vi "反控数据上传(子VI).vi"(11 "QN":string) -> ()   [LabVIEW 2016, in "数据传输系统.lvlib"]
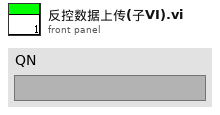
[diagram p1: front panel]
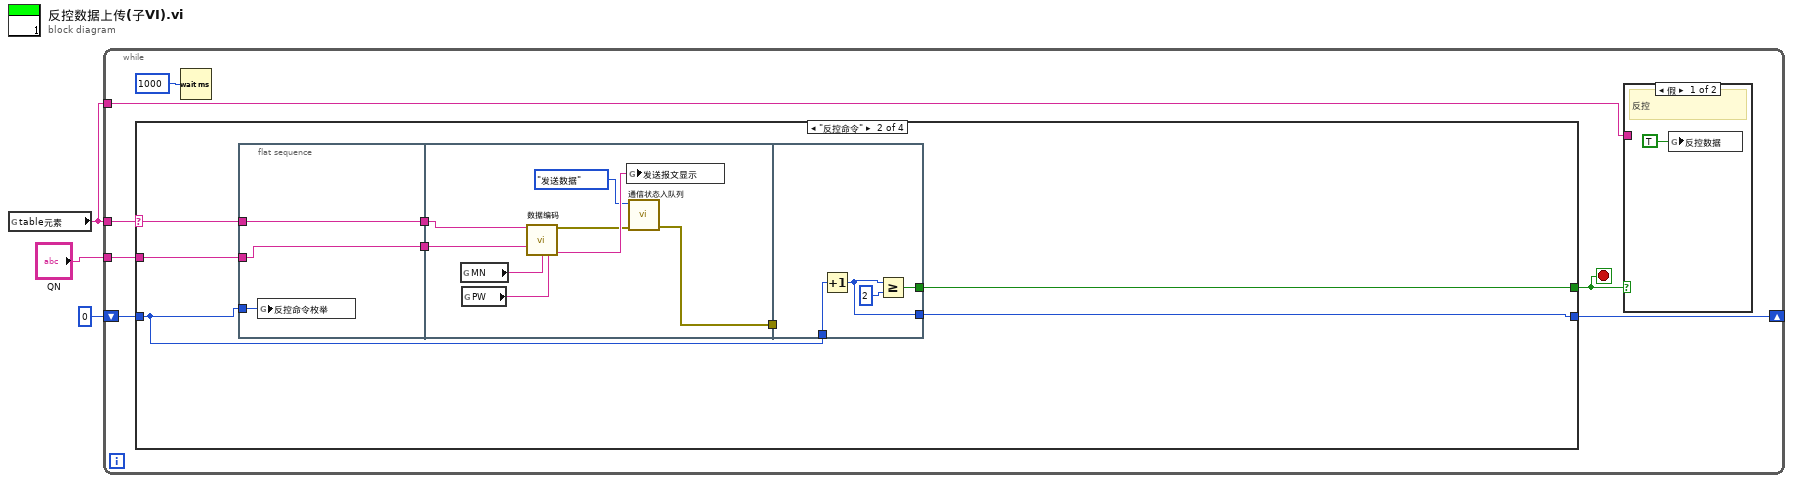
[diagram p0: block diagram]
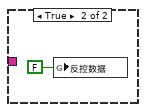
[diagram p2: hidden frame]
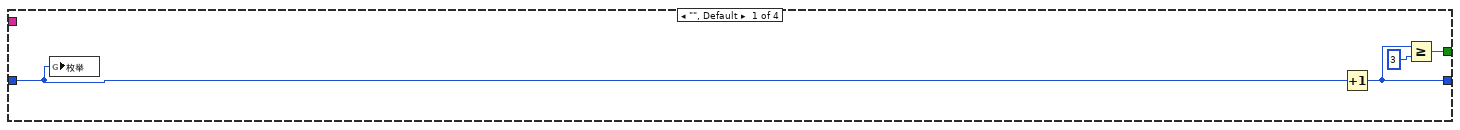
[diagram p3: hidden frame]
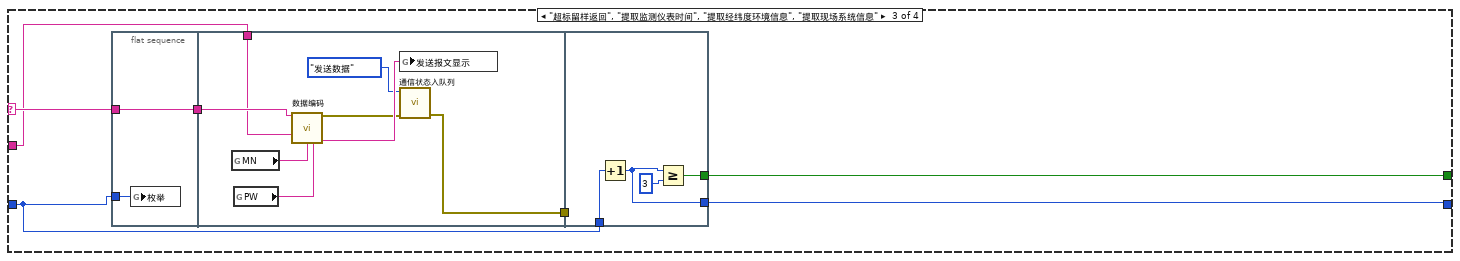
[diagram p4: hidden frame]
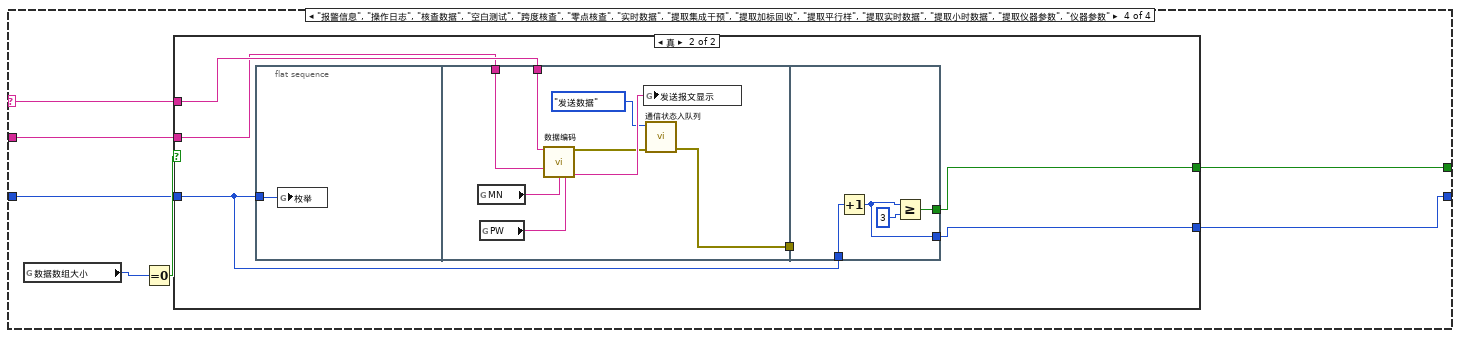
[diagram p5: hidden frame]
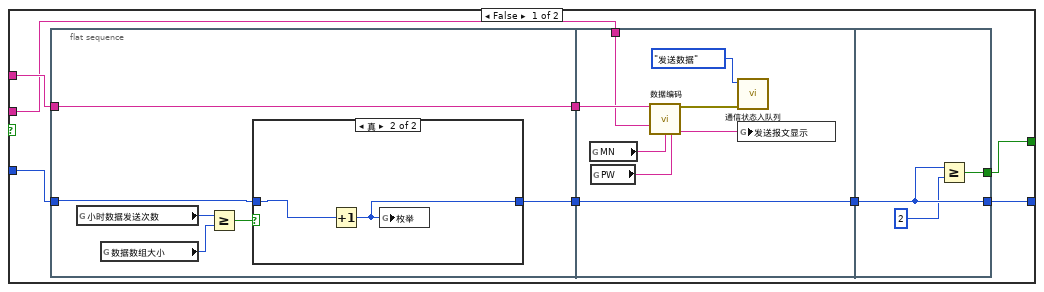
[diagram p6: hidden frame]
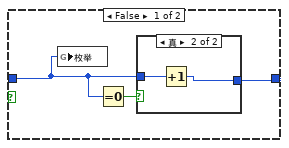
[diagram p7: hidden frame]
diagram:
  n1 = global read "全局1.vi" "table元素"() -> (w3:string)
  n2 = while {
    tunnel: w3 -> [w10]
    shift-right: [w8] -> _
    shift-left: 0 -> [w9]
    tunnel: w3 -> [w6]
    tunnel: "QN" -> [w4]
    stop <- w7 stop-if-true
    n3 = case shown="\"反控命令\"" w10 {
      selector: w10 -> [_ w21 w46 w63]
      tunnel: w9 -> [w15 w22 w43 w62]
      tunnel: [w14 w19 w42 w67] -> w7
      tunnel: [w13 w20 w41 w66] -> w8
      tunnel: w4 -> [_ w18 w40 w61]
      frame "", Default {
        n4 = global write "全局1.vi" "枚举"(w15) -> ()
        n5 = Increment(x=w15) -> (x+1=w13:i32)
        n6 = Greater Or Equal?(x=w13, y=3) -> (x >= y?=w14:bool)
      }
      frame "反控命令" {
        n7 = flat-sequence {
          tunnel: w21 -> [w27]
          tunnel: [w27] -> w24
          tunnel: w22 -> [w26]
          tunnel: w18 -> [w25]
          tunnel: [w25] -> w17
          tunnel: w24 -> [w30]
          tunnel: [w29] -> w23
          tunnel: w17 -> [w28]
          tunnel: w23 -> [_]
          tunnel: w22 -> [w38]
          tunnel: [w37] -> w19
          tunnel: [w36] -> w20
          frame #0 {
            n8 = global write "全局 反控命令枚举.vi" "反控命令枚举"(w26) -> ()
          }
          frame #1 {
            n9 = global read "断电保存全局.vi" "MN"() -> (w35:string)
            n10 = global read "断电保存全局.vi" "PW"() -> (w34:string)
            n11 = call "数据编码.vi"("table输入"=w30, "QN"=w28, "MN"=w35, "PW"=w34) -> ("错误常量"=w32:errorcluster, "通讯包字符串"=w33:string)  [unwired: 10 in]
            n12 = global write "全局1.vi" "发送报文显示"(w33) -> ()
            n13 = call "通信状态入队列.vi"("错误输入（无错误）"=w32, "枚举"=enum16{"打开连接", "发送数据", "读取数据", "数据处理", "关闭连接"}."发送数据") -> ("错误输出"=w29:errorcluster)  [unwired: 9 in]
          }
          frame #2 {
            n14 = Increment(x=w38) -> (x+1=w36:i32)
            n15 = Greater Or Equal?(x=w36, y=2) -> (x >= y?=w37:bool)
          }
        }
      }
      frame "超标留样返回", "提取监测仪表时间", "提取经纬度环境信息", "提取现场系统信息" {
        n16 = flat-sequence {
          tunnel: w46 -> [w48]
          tunnel: [w48] -> w45
          tunnel: w43 -> [w47]
          tunnel: w45 -> [w51]
          tunnel: [w50] -> w44
          tunnel: w40 -> [w49]
          tunnel: w44 -> [_]
          tunnel: w43 -> [w59]
          tunnel: [w58] -> w42
          tunnel: [w57] -> w41
          frame #0 {
            n17 = global write "全局1.vi" "枚举"(w47) -> ()
          }
          frame #1 {
            n18 = global read "断电保存全局.vi" "MN"() -> (w56:string)
            n19 = global read "断电保存全局.vi" "PW"() -> (w55:string)
            n20 = call "数据编码.vi"("table输入"=w51, "QN"=w49, "MN"=w56, "PW"=w55) -> ("错误常量"=w53:errorcluster, "通讯包字符串"=w54:string)  [unwired: 10 in]
            n21 = global write "全局1.vi" "发送报文显示"(w54) -> ()
            n22 = call "通信状态入队列.vi"("错误输入（无错误）"=w53, "枚举"=enum16{"打开连接", "发送数据", "读取数据", "数据处理", "关闭连接"}."发送数据") -> ("错误输出"=w50:errorcluster)  [unwired: 9 in]
          }
          frame #2 {
            n23 = Increment(x=w59) -> (x+1=w57:i32)
            n24 = Greater Or Equal?(x=w57, y=3) -> (x >= y?=w58:bool)
          }
        }
      }
      frame "报警信息", "操作日志", "核查数据", "空白测试", "跨度核查", "零点核查", "实时数据", "提取集成干预", "提取加标回收", "提取平行样", "提取实时数据", "提取小时数据", "提取仪器参数", "仪器参数" {
        n25 = global read "全局 数据数组大小.vi" "数据数组大小"() -> (w65:i32)
        n26 = Equal To 0?(x=w65) -> (x = 0?=w64:bool)
        n27 = case shown="真" w64 {
          tunnel: [w72 w102] -> w67
          tunnel: [w71 w103] -> w66
          tunnel: w63 -> [w70 w105]
          tunnel: w62 -> [w69 w104]
          tunnel: w61 -> [w68 w101]
          frame False {
            n28 = flat-sequence {
              tunnel: w69 -> [w78]
              tunnel: [w76] -> w75
              tunnel: w70 -> [w77]
              tunnel: [w77] -> w74
              tunnel: w75 -> [w97]
              tunnel: [w97] -> w73
              tunnel: w74 -> [w91]
              tunnel: w68 -> [w90]
              tunnel: w73 -> [w100]
              tunnel: [w100] -> w71
              tunnel: [w99] -> w72
              frame #0 {
                n29 = global read "全局 小时数据发送次数.vi" "小时数据发送次数"() -> (w80:i32)
                n30 = global read "全局 数据数组大小.vi" "数据数组大小"() -> (w81:i32)
                n31 = Greater Or Equal?(x=w80, y=w81) -> (x >= y?=w79:bool)
                n32 = case shown="真" w79 {
                  tunnel: w78 -> [w83 w89]
                  tunnel: [w84 w88] -> w76
                  frame False {
                    n33 = global write "全局1.vi" "枚举"(w83) -> ()
                    n34 = Equal To 0?(x=w83) -> (x = 0?=w82:bool)
                    n35 = case shown="真" w82 {
                      tunnel: w83 -> [w85 w87]
                      tunnel: [w85 w86] -> w84
                      frame False {
                      }
                      frame True {
                        n36 = Increment(x=w87) -> (x+1=w86:i32)
                      }
                    }
                  }
                  frame True {
                    n37 = Increment(x=w89) -> (x+1=w88:i32)
                    n38 = global write "全局1.vi" "枚举"(w88) -> ()
                  }
                }
              }
              frame #1 {
                n39 = global read "断电保存全局.vi" "MN"() -> (w92:string)
                n40 = global read "断电保存全局.vi" "PW"() -> (w93:string)
                n41 = call "数据编码.vi"("table输入"=w91, "QN"=w90, "MN"=w92, "PW"=w93) -> ("错误常量"=w95:errorcluster, "通讯包字符串"=w94:string)  [unwired: 10 in]
                n42 = call "通信状态入队列.vi"("错误输入（无错误）"=w95, "枚举"=enum16{"打开连接", "发送数据", "读取数据", "数据处理", "关闭连接"}."发送数据") -> ()  [unwired: 9 in, 1 out]
                n43 = global write "全局1.vi" "发送报文显示"(w94) -> ()
              }
              frame #2 {
                n44 = Greater Or Equal?(x=w100, y=2) -> (x >= y?=w99:bool)
              }
            }
          }
          frame True {
            n45 = flat-sequence {
              tunnel: w104 -> [w107]
              tunnel: [w110] -> w106
              tunnel: w105 -> [w109]
              tunnel: w101 -> [w108]
              tunnel: w106 -> [_]
              tunnel: [w118] -> w102
              tunnel: [w117] -> w103
              tunnel: w104 -> [w116]
              frame #0 {
                n46 = global write "全局1.vi" "枚举"(w107) -> ()
              }
              frame #1 {
                n47 = global read "断电保存全局.vi" "MN"() -> (w115:string)
                n48 = global read "断电保存全局.vi" "PW"() -> (w114:string)
                n49 = call "数据编码.vi"("table输入"=w109, "QN"=w108, "MN"=w115, "PW"=w114) -> ("错误常量"=w112:errorcluster, "通讯包字符串"=w113:string)  [unwired: 10 in]
                n50 = global write "全局1.vi" "发送报文显示"(w113) -> ()
                n51 = call "通信状态入队列.vi"("错误输入（无错误）"=w112, "枚举"=enum16{"打开连接", "发送数据", "读取数据", "数据处理", "关闭连接"}."发送数据") -> ("错误输出"=w110:errorcluster)  [unwired: 9 in]
              }
              frame #2 {
                n52 = Increment(x=w116) -> (x+1=w117:i32)
                n53 = Greater Or Equal?(x=w117, y=3) -> (x >= y?=w118:bool)
              }
            }
          }
        }
      }
    }
    n54 = Wait (ms)(milliseconds to wait=u32 1000 ("等待时间（毫秒）")) -> ()  [unwired: 1 out]
    n55 = case shown="假" w7 {
      tunnel: w6 -> [_ _]
      frame False {
        # "反控"
        n56 = global write "全局1.vi" "反控数据"(TRUE ("反控数据")) -> ()
      }
      frame True {
        n57 = global write "全局1.vi" "反控数据"(FALSE ("反控数据")) -> ()
      }
    }
  }
